vi "TDMS_test.vi"() -> ()   [LabVIEW 2018]
panel:
  out "Full time, ms":u32
  out "time to run 1 cycle, ms":dbl
  in  "file path":path=path "C:/Users/Dmitriy/Documents/MHC_Tracker/test.tdms"
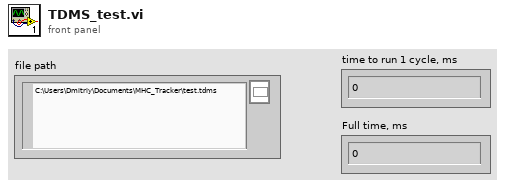
[diagram p1: front panel]
types:
  T1 = enum16{"open", "open or create", "create or replace", "create", "open (read-only)"}
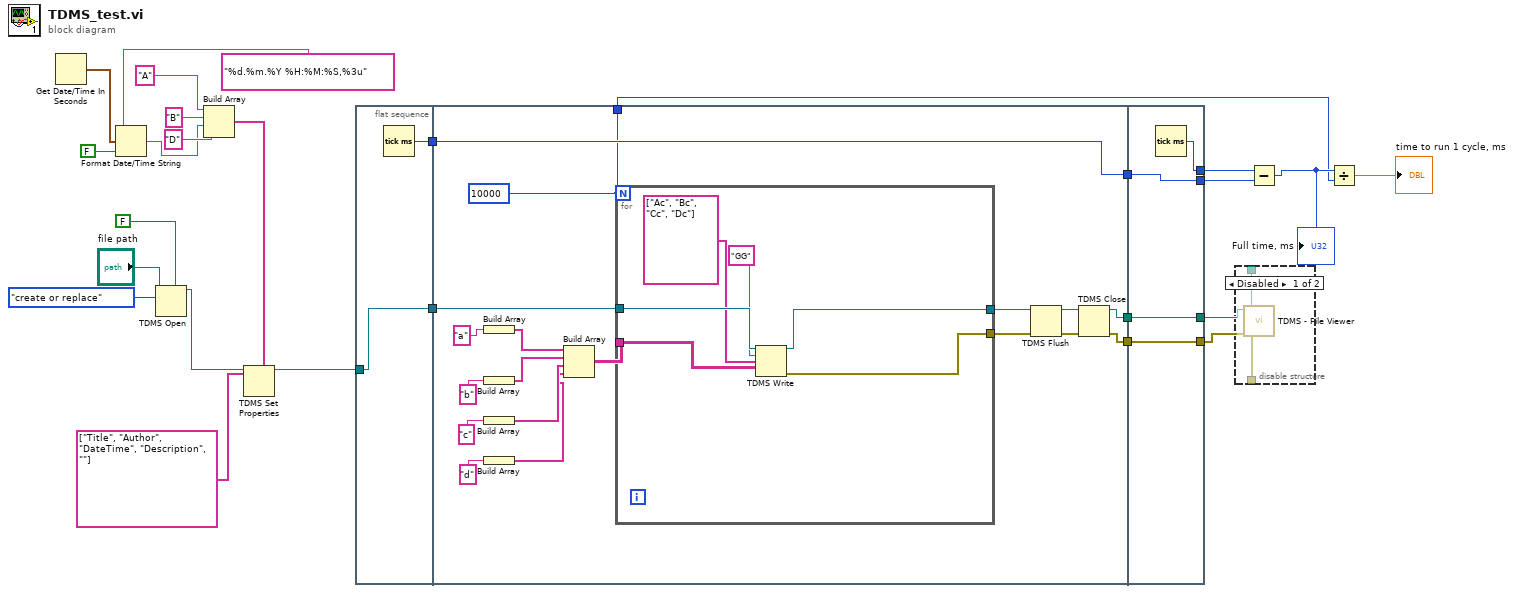
[diagram p0: block diagram]
diagram:
  n1 = Get Date/Time In Seconds() -> (seconds since 1Jan1904=w3:timestamp)
  n2 = Format Date/Time String(time format string (%c)="%d.%m.%Y %H:%M:%S,%3u" ("format string"), seconds (now)=w3, UTC format=FALSE) -> (date/time string=w4:string)
  n3 = TDMS Open(5:FALSE ("create index file? (T)"), 10:T1."create or replace" ("operation (0:open)"), 11:"file path") -> (3:w9:refnum<k34>)  [unwired: 4 in, 1 out]
  n4 = Build Array("A", "B" ("element"), w4, "D" ("element")) -> (w2:string[])
  n5 = TDMS Set Properties(5:w2, 7:string[] ["Title", "Author", "DateTime", "Description", ""] ("property names"), 11:w9) -> (3:w11:refnum<k34>)  [unwired: 3 in, 3 out]
  n6 = flat-sequence {
    tunnel: [w27] -> w24
    tunnel: [w28] -> w18
    tunnel: w11 -> [w27]
    tunnel: w24 -> [w31]
    tunnel: [w44] -> w23
    tunnel: [w43] -> w22
    tunnel: [w42] -> w19
    tunnel: w18 -> [w42]
    tunnel: [w41] -> w16
    tunnel: [w55] -> w13
    tunnel: [w56] -> w14
    tunnel: w23 -> [w56]
    tunnel: w22 -> [w55]
    tunnel: [w54] -> w21
    tunnel: [w53] -> w20
    tunnel: w19 -> [w53]
    frame #0 {
      n7 = Tick Count (ms)() -> (millisecond timer value=w28:u32)
    }
    frame #1 {
      w41 = 10000
      n8 = Build Array("a") -> (w40:string[])
      n9 = Build Array("b") -> (w38:string[])
      n10 = Build Array("c") -> (w37:string[])
      n11 = Build Array("d") -> (w36:string[])
      n12 = Build Array(w40, w38, w37, w36) -> (w39:string[][])
      n13 = for {
        N: w41 -> [_]
        tunnel: w39 -> [w49]
        tunnel: w31 -> [w52]
        tunnel: [w51] -> w30
        tunnel: [w50] -> w29
        n14 = TDMS Write(0:w52, 5:"GG" ("group name in (Untitled)"), 7:string[] ["Ac", "Bc", "Cc", "Dc"], 9:w49) -> (4:w51:refnum<k34>, 15:w50:errorcluster)  [unwired: 2 in, 2 out]
      }
      n15 = TDMS Flush(4:w29, 7:w30) -> (0:w46:errorcluster, 3:w45:refnum<k34>)
      n16 = TDMS Close(8:w46, 11:w45) -> (0:w43:errorcluster, 3:w44:path)
    }
    frame #2 {
      n17 = Tick Count (ms)() -> (millisecond timer value=w54:u32)
    }
  }
  n18 = disable-structure shown="Disabled" {
    disable-tunnel: w14 -> [w58 _]
    disable-tunnel: w13 -> [w57 _]
    frame Disabled {
      n19 = call <vilib>:"TDMS - File Viewer.vi"("error in (no error)"=w57, "file path"=w58) -> ()  [unwired: 4 in, 2 out]
    }
    frame Enabled {
    }
  }
  n20 = Subtract(x=w21, y=w20) -> (x-y=w17:u32)
  "Full time, ms" <- w17
  n21 = Divide(x=w17, y=w16) -> (x/y=→"time to run 1 cycle, ms":dbl)
